vi "tcs shm get Sample kernel Optics Vt LV.vi"(8 "error in (no error)":errorcluster, 11 "kernel_OpticsVt_Ctl":cluster{"tilt":sgl, "tip":sgl}) -> (0 "error out":errorcluster, 2 "function return":i32, 3 "kernel_OpticsVt_Ctl out":cluster{"tilt":sgl, "tip":sgl})   [LabVIEW 2016, in "SALLV_tcs.lvlib"]
doc: "int tcs_shm_getSample_kernel_OpticsVtLV(tcs_kernel_OpticsVtLV *kernel_OpticsVt_Ctl );"
uses:
  SALLV_tcs.lvlib
  SALLV_tcs.so
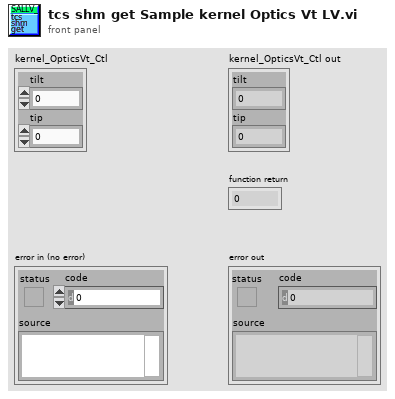
[diagram p1: front panel]
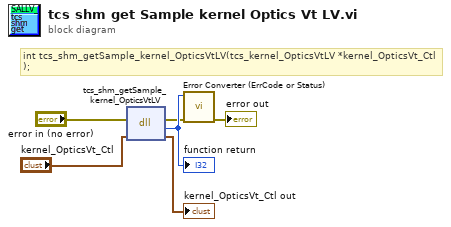
[diagram p0: block diagram]
diagram:
  # "int tcs_shm_getSample_kernel_OpticsVtLV(tcs_kernel_OpticsVtLV *kernel_OpticsVt_Ctl );"
  n1 = dll-call lib="home/andres/Desktop/SALLV_tcs/SALLV_tcs.*" fn="tcs_shm_getSample_kernel_OpticsVtLV"(error in="error in (no error)", "kernel_OpticsVt_Ctl"="kernel_OpticsVt_Ctl") -> (error out=w2:errorcluster, w6:i32, "kernel_OpticsVt_Ctl"=→"kernel_OpticsVt_Ctl out":cluster{"tilt":sgl, "tip":sgl})  [unwired: 2 in, 1 out]
  "function return" <- w6
  n2 = call "Error Converter (ErrCode or Status).vi"("error in (no error)"=w2, "error code"=w6) -> ("error out"=→"error out":errorcluster)  [unwired: 9 in]
